vi "setChannel.vi"(8 "error in (no error)":errorcluster, 10 "Channel.lvclass":refnum<class "Channel.lvclass">, 11 "SingleToneRamp.lvclass in":refnum<class "SingleToneRamp.lvclass">) -> (0 "error out":errorcluster, 3 "SingleToneRamp.lvclass out":refnum<class "SingleToneRamp.lvclass">)   [LabVIEW 2011, in "Tools.lvlib" / "Scripting.lvlib" / "SingleToneRamp.lvclass"]
uses:
  SingleToneRamp.lvclass
  DatabaseHelpers/Database Objects/Channel/Channel.lvclass
  SingleTone.lvclass
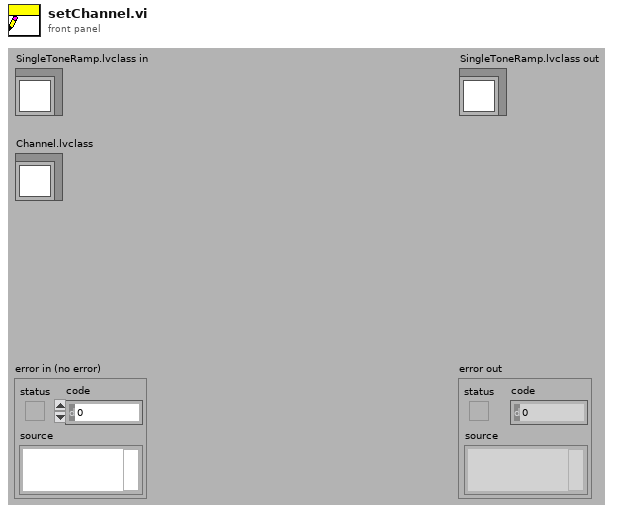
[diagram p1: front panel]
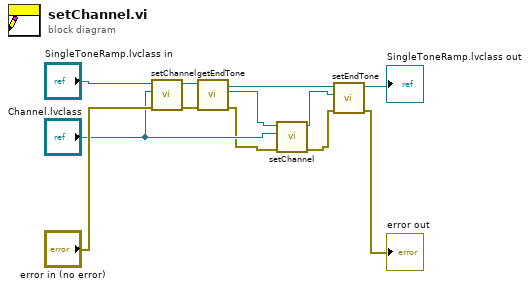
[diagram p0: block diagram]
diagram:
  n1 = call-parent "setChannel.vi"("error in (no error)"="error in (no error)", "Channel.lvclass"="Channel.lvclass", "ScriptEvent.lvclass in"="SingleToneRamp.lvclass in") -> ("error out"=w7:errorcluster, "ScriptEvent.lvclass out"=w9:refnum<class "SingleToneRamp.lvclass">)  [unwired: 7 in]
  n2 = call "getEndTone.vi"("error in (no error)"=w7, "SingleToneRamp.lvclass in"=w9) -> ("error out"=w3:errorcluster, "endTone"=w5:refnum<class "SingleTone.lvclass">, "SingleToneRamp.lvclass out"=w10:refnum<class "SingleToneRamp.lvclass">)  [unwired: 7 in]
  n3 = call-dynamic "setChannel.vi"("error in (no error)"=w3, "Channel.lvclass"="Channel.lvclass", "ScriptEvent.lvclass in"=w5) -> ("error out"=w2:errorcluster, "ScriptEvent.lvclass out"=w1:refnum<class "SingleTone.lvclass">)  [unwired: 7 in]
  n4 = call "setEndTone.vi"("error in (no error)"=w2, "EndTone"=w1, "SingleToneRamp.lvclass in"=w10) -> ("error out"=→"error out":errorcluster, "SingleToneRamp.lvclass out"=→"SingleToneRamp.lvclass out":refnum<class "SingleToneRamp.lvclass">)  [unwired: 7 in]
